vi "Write Table Data.vi"(8 "error in":errorcluster, 10 "Value":string[][](array[string]), 11 "Table Ref in":refnum<vi>) -> (0 "error out":errorcluster, 3 "Table Ref out":refnum<vi>)   [LabVIEW 2020, in "G-Unicode.lvlib"]
uses:
  G-Unicode.lvlib
  Unicode/Controls/String Encoding.ctl
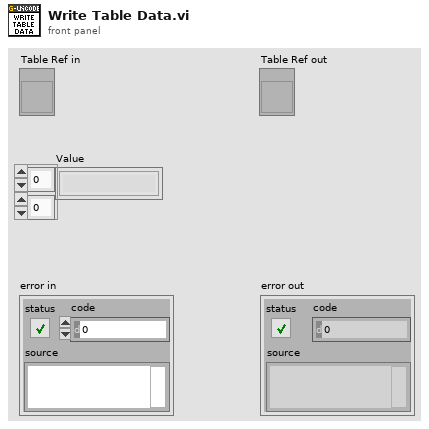
[diagram p1: front panel]
types:
  T1 = typedef "G-Unicode.lvlib/String Encoding.ctl" = enum16{"ANSI", "UTF-8", "UTF-16LE", "UTF-16BE", "Unknown"}
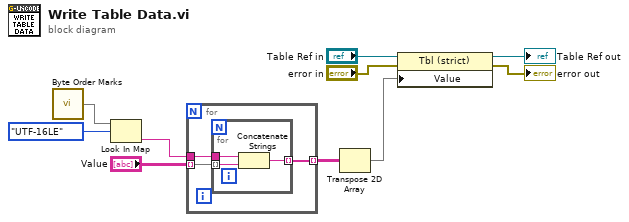
[diagram p0: block diagram]
diagram:
  n1 = call "Byte Order Marks.vi"() -> ("BOMs"=w3:map{T1, string})
  n2 = Look In Map(map=w3, key=String_Encoding."UTF-16LE") -> (value=w1:string)  [unwired: 1 in, 1 out]
  n3 = for {
    tunnel: "Value" -> [w13] mode=indexing
    tunnel: [w12] -> w5 mode=indexing
    tunnel: w1 -> [w11]
    n4 = for {
      tunnel: w13 -> [w16] mode=indexing
      tunnel: [w15] -> w12 mode=indexing
      tunnel: w11 -> [w14]
      n5 = Concatenate Strings(w14, w16) -> (w15:string)
    }
  }
  n6 = Transpose 2D Array(2D array=w5) -> (transposed array=w4:string[][])
  n7 = property class="Tbl (strict)"(reference="Table Ref in", error in="error in", "Value"=w4) -> (reference out=→"Table Ref out":refnum<vi>, error out=→"error out":errorcluster)
